vi "Add Routing and Faulting Custom Device.vi"(8 "error in":errorcluster, 11 "target in":refnum<k24>) -> (0 "error out":errorcluster, 2 "routing and faulting custom device":T1 format="%.0x", 3 "target out":refnum<k24>)   [LabVIEW 2020, in "Routing and Faulting Scripting.lvlib"]
doc: "Creates and adds a new instance of the Routing and Faulting custom device to the target."
uses:
  Routing and Faulting Scripting.lvlib
  NationalInstruments.VeriStand.SystemDefinitionAPI
  <vilib>/NI VeriStand/Custom Device API/Custom Device Item Ref.ctl
  Shared/Constants.vi
  Dependencies.llb/Routing and Faulting Shared.lvlib
  <vilib>/NI VeriStand/Custom Device API/Custom Device API.lvlib
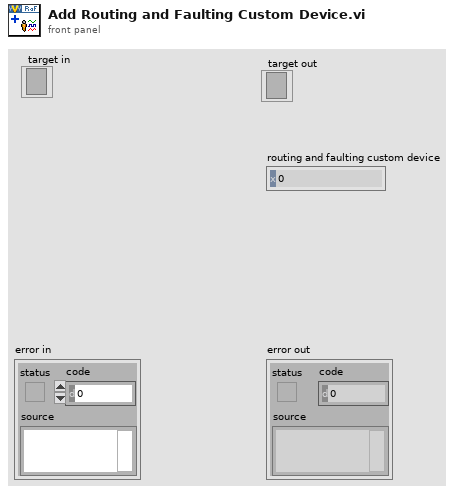
[diagram p1: front panel]
types:
  T1 = typedef "Custom Device API.lvlib/Custom Device Item Ref.ctl" = u64
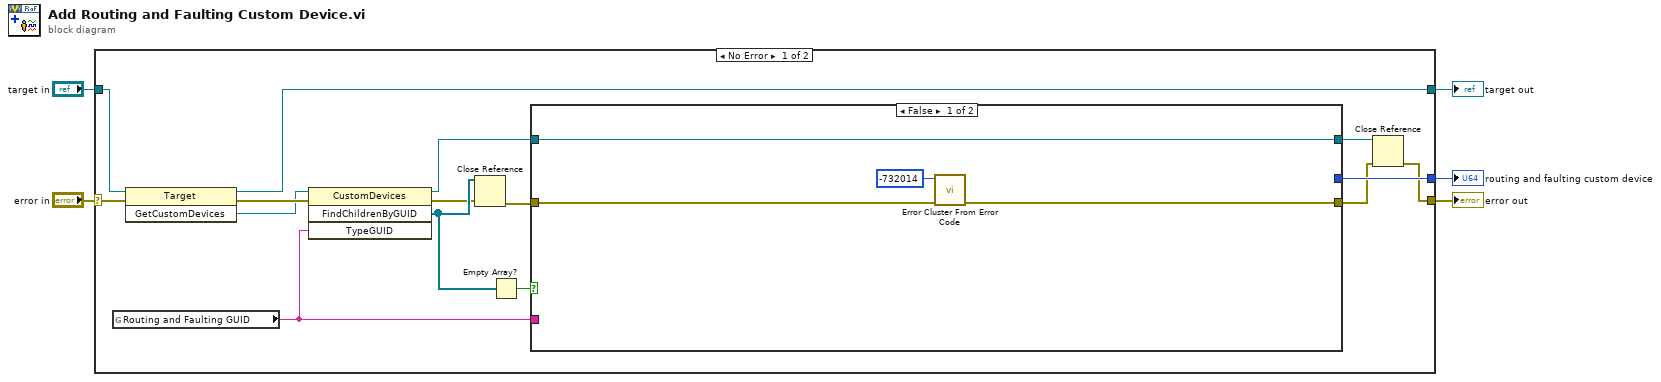
[diagram p0: block diagram]
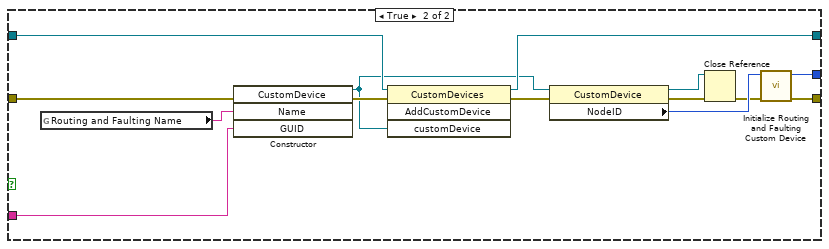
[diagram p2: hidden frame]
diagram:
  n1 = case shown="No Error" "error in" {
    selector: "error in" -> [w7 w40]
    tunnel: [w11 w40] -> w5
    tunnel: "target in" -> [w8 w39]
    tunnel: [w20 w39] -> w2
    tunnel: [w19 _] -> w1
    frame No Error {
      n2 = global read "Constants.vi" "Routing and Faulting GUID"() -> (w6:string)
      n3 = invoke class="Target" method="GetCustomDevices"(reference=w8, error in=w7) -> (reference out=w20:refnum<k24>, error out=w17:errorcluster, "GetCustomDevices"=w10:refnum<k24>)  [unwired: 1 in]
      n4 = invoke class="CustomDevices" method="FindChildrenByGUID"(reference=w10, error in=w17, "TypeGUID"=w6) -> (reference out=w9:refnum<k24>, error out=w15:errorcluster, "FindChildrenByGUID"=w16:refnum<k24>[])  [unwired: 1 in, 1 out]
      n5 = Close Reference(reference=w16, error in (no error)=w15) -> (error out=w14:errorcluster)
      n6 = Empty Array?(array=w16) -> (empty?=w18:bool)
      n7 = case shown="False" w18 {
        tunnel: [w22 w35] -> w12
        tunnel: [_ w34] -> w19
        tunnel: w9 -> [w24 w29]
        tunnel: w14 -> [w21 w27]
        tunnel: [w24 w28] -> w13
        tunnel: w6 -> [_ w25]
        frame False {
          n8 = call <vilib>:"Error Cluster From Error Code.vi"("error in (no error)"=w21, "error code (0)"=-732014) -> ("error out"=w22:errorcluster)  [unwired: 7 in]
        }
        frame True {
          n9 = global read "Constants.vi" "Routing and Faulting Name"() -> (w30:string)
          n10 = constructor class="CustomDevice"(error in=w27, "Name"=w30, "GUID"=w25) -> (reference out=w26:refnum<k24>, error out=w38:errorcluster)  [unwired: 2 in, 3 out]
          n11 = invoke class="CustomDevices" method="AddCustomDevice"(reference=w29, error in=w38, "customDevice"=w26) -> (reference out=w28:refnum<k24>, error out=w37:errorcluster)  [unwired: 1 in, 2 out]
          n12 = property class="CustomDevice"(reference=w26, error in=w37) -> (reference out=w33:refnum<k24>, error out=w32:errorcluster, "NodeID"=w36:u64)
          n13 = Close Reference(reference=w33, error in (no error)=w32) -> (error out=w31:errorcluster)
          n14 = call "Initialize Routing and Faulting Custom Device.vi"("error in"=w31, "routing and faulting custom device in"=w36) -> ("error out"=w35:errorcluster, "routing and faulting custom device out"=w34:T1)  [unwired: 6 in, 2 out]
        }
      }
      n15 = Close Reference(reference=w13, error in (no error)=w12) -> (error out=w11:errorcluster)
    }
    frame Error {
    }
  }
  "target out" <- w2
  "error out" <- w5
  "routing and faulting custom device" <- w1
